vi "S7Ref.vi"() -> ()   [LabVIEW 2020]
panel:
  in  "TCP句柄 2":refnum<k5>
  in  "S7Ref":refnum<k5>
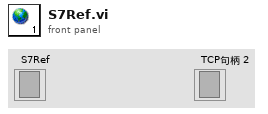
[diagram p1: front panel]
diagram:
